vi "Sell product.vi"(8 "error in (no error)":errorcluster, 11 "Data Cluster":T1) -> (0 "error out":errorcluster)   [LabVIEW 2019, in "Products.lvlib"]
uses:
  Products.lvlib
  Module Data--cluster.ctl
  Mensajes/Messages.lvlib
  Monedas/Monedas.lvlib
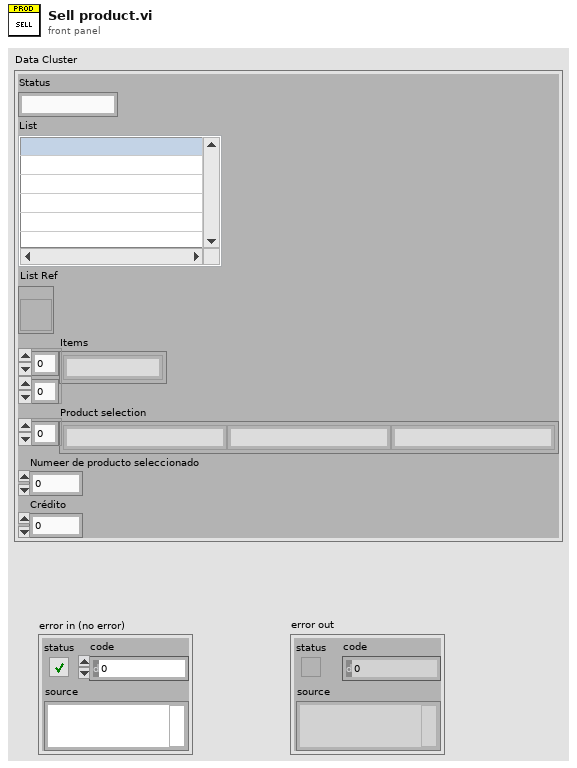
[diagram p1: front panel]
types:
  T1 = typedef "Products.lvlib/Module Data--cluster.ctl" = cluster{"Status":string, "List":i32, "List Ref":refnum<vi>, "Items":string[][], "Product selection":string[], "Numeer de producto seleccionado":i32, "Crédito":dbl}
  T2 = typedef "Monedas.lvlib/Request_Crédito (Reply Payload)--cluster.ctl" = cluster{"Crédito":dbl, "Request_Crédito_error":errorcluster}
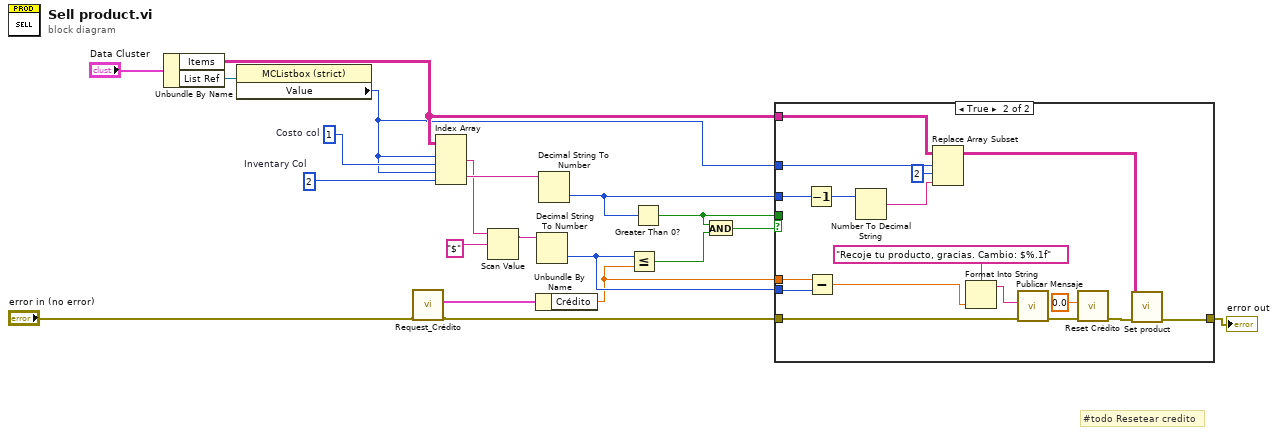
[diagram p0: block diagram]
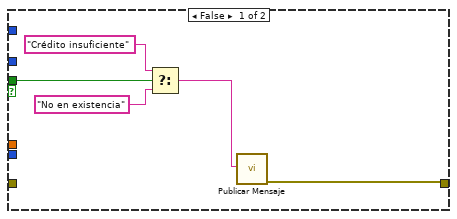
[diagram p2: hidden frame]
diagram:
  w18 = 2  # Inventary Col
  w19 = 1  # Costo col
  # "#todo Resetear credito"
  n1 = Unbundle By Name("Data Cluster") -> ("Items"=w11:string[][], "List Ref"=w20:refnum<vi>)
  n2 = property class="MCListbox (strict)"(reference=w20) -> ("Value"=w10:i32)  [unwired: 1 in, 2 out]
  n3 = call "Request_Crédito.vi"("error in (no error)"="error in (no error)") -> ("error out"=w2:errorcluster, "Reply Payload"=w1:T2)  [unwired: 8 in, 1 out]
  n4 = Index Array(array=w11, index (row) #1=w10, index (col) #1=w19, index (row) #2=w10, index (col) #2=w18) -> (element #1=w5:string, element #2=w17:string)
  n5 = Scan Value(string=w5, format string="$" ("input string")) -> (output string=w4:string)  [unwired: 1 in, 1 out]
  n6 = Unbundle By Name(w1) -> ("Crédito"=w13:dbl)
  n7 = Decimal String To Number(string=w4) -> (number=w14:i32)  [unwired: 2 in, 1 out]
  n8 = Decimal String To Number(string=w17) -> (number=w12:i32)  [unwired: 2 in, 1 out]
  n9 = Less Or Equal?(x=w14, y=w13) -> (x <= y?=w16:bool)
  n10 = Greater Than 0?(x=w12) -> (x > 0?=w8:bool)
  n11 = And(x=w8, y=w16) -> (x .and. y?=w15:bool)
  n12 = case shown="True" w15 {
    tunnel: w14 -> [_ w42]
    tunnel: w13 -> [_ w41]
    tunnel: w12 -> [_ w40]
    tunnel: w11 -> [_ w38]
    tunnel: w10 -> [_ w37]
    tunnel: [w24 w33] -> w9
    tunnel: w8 -> [w25 _]
    tunnel: w2 -> [_ w29]
    frame False {
      n13 = Select(t="Crédito insuficiente", s=w25, f="No en existencia") -> (s? t:f=w23:string)
      n14 = call "Publicar Mensaje.vi"("Mensaje"=w23) -> ("error out"=w24:errorcluster)  [unwired: 10 in]
    }
    frame True {
      n15 = Decrement(x=w40) -> (x-1=w39:i32)
      n16 = Subtract(x=w41, y=w42) -> (x-y=w30:dbl)
      n17 = Number To Decimal String(number=w39) -> (decimal integer string=w35:string)  [unwired: 1 in]
      n18 = Replace Array Subset(array=w38, new element=w35, index (row)=w37, index (col)=2 ("disabled index (col)")) -> (w34:string[][])
      n19 = Format Into String(format string="Recoje tu producto, gracias. Cambio: $%.1f", w30) -> (resulting string=w32:string)  [unwired: 2 in, 1 out]
      n20 = call "Publicar Mensaje.vi"("error in (no error)"=w29, "Mensaje"=w32) -> ("error out"=w28:errorcluster)  [unwired: 9 in]
      n21 = call "Reset Crédito.vi"("error in (no error)"=w28, "Crédito"=0.0) -> ("error out"=w27:errorcluster)  [unwired: 9 in]
      n22 = call "Set product.vi"("error in (no error)"=w27, "Item Names"=w34) -> ("error out"=w33:errorcluster)  [unwired: 9 in]
    }
  }
  "error out" <- w9
